vi "Practica_3.vi"() -> ()   [LabVIEW 2016]
uses:
  Control_1Enum.ctl
panel:
  out "String":string
  out "unsigned 8bit integer":u8
  out "Tab Control":T1(tab)
  out "Anuncios":u8(ring)
  in  "Boton_Aceptar_Contrasena":bool
  in  "Contrasena":string
  in  "Salir":bool
  out "Adeudo_Tarjeta":dbl
  out "Credito_Disponible":dbl
  in  "Estado_de_cuenta":bool
  in  "Depositos_otras_cuentas":bool
  in  "Donativos":bool
  in  "Compra_Tiempo_Aire":bool
  in  "Pago_Tarjeta_Credito":bool
  in  "Retirar Efectivo":bool
  in  "Regresar_1":bool
  in  "Retirar Efectivo 2":bool
  in  "Cantidad_a_Retirar":dbl min=0.0 max=10000.0
  out "Adeudo_Tarjeta 2":dbl
  out "Credito_Disponible 2":dbl
  in  "Regresar_2":bool
  in  "Monto_a_Pagar":dbl min=0.0 max=10000.0
  in  "Pago_Tarjeta_Credito 2":bool
  out "Adeudo_Tarjeta 3":dbl
  out "Credito_Disponible 3":dbl
  in  "Regresar_3":bool
  out "Adeudo_Tarjeta 4":dbl
  out "Credito_Disponible 4":dbl
  in  "Recargar_100":bool
  in  "Recargar_200":bool
  in  "Recargar_300":bool
  in  "Recargar_500":bool
  in  "Regresar_4":bool
  out "Adeudo_Tarjeta 5":dbl
  out "Credito_Disponible 5":dbl
  in  "Donar_100":bool
  in  "Donar_200":bool
  in  "Donar_300":bool
  in  "Donar_500":bool
  in  "Combo Box":string(combo)="World Vision Mexico"
  in  "Regresar_5":bool
  in  "Boton_Punto":bool
  out "String 2":string
  in  "Combo Box 2":string(combo)="Adrian Barba"
  out "Adeudo_Tarjeta 6":dbl
  out "Credito_Disponible 6":dbl
  in  "Boton_Aceptar":bool
  in  "Boton_Borrar":bool
  in  "Boton_9":bool
  in  "Boton_Limpiar":bool
  in  "Boton_6":bool
  in  "Boton_0":bool
  in  "Boton_3":bool
  in  "Boton_8":bool
  in  "Boton_7":bool
  in  "Boton_5":bool
  in  "Boton_4":bool
  in  "Boton_2":bool
  in  "Boton_1":bool
  in  "Regresar_6":bool
  out "Transacciones":string
  in  "Tarjeta":bool
  out "Led_Parpadeante":bool
  # "INGRESE SU CLAVE"
  # "Contraseña"
  # "Operaciones a Realizar"
  # "Retirar Credito"
  # "Pagar la Tarjeta"
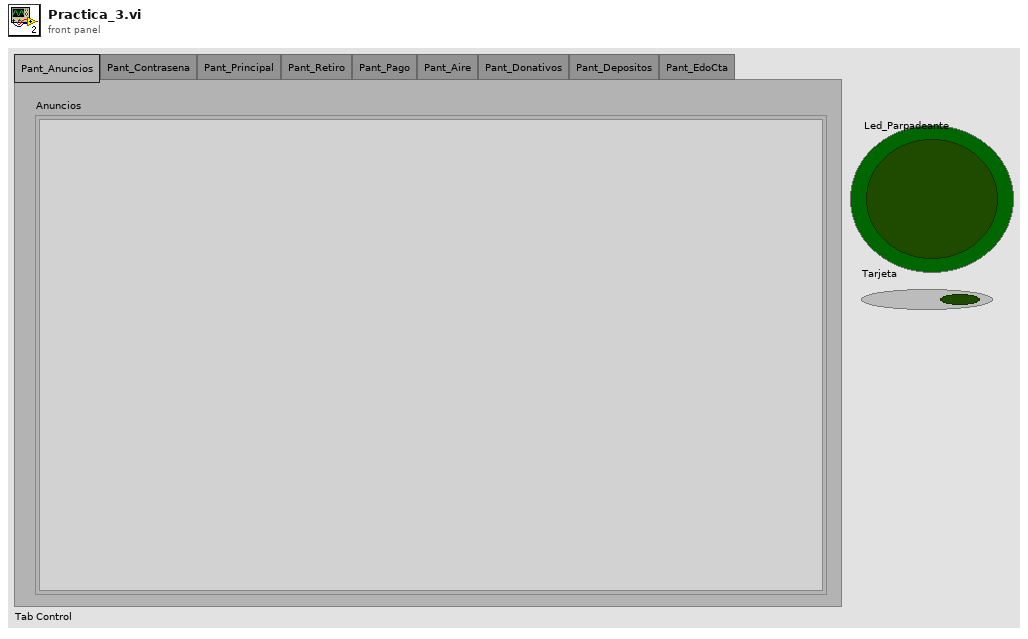
[diagram p1: front panel]
types:
  T1 = enum32{"Pant_Anuncios", "Pant_Contrasena", "Pant_Principal", "Pant_Retiro", "Pant_Pago", "Pant_Aire", "Pant_Donativos", "Pant_Depositos", "Pant_EdoCta"}
  T2 = typedef "Control_1Enum.ctl" = enum16{"Inicio", "Preguntar_Usuario", "Contrasena_valida", "Menu_Principal", "Menu_Retiro", "Menu_Pago", "Compra_TAire", "Donativos", "Depositos", "Estado_Cuenta"}
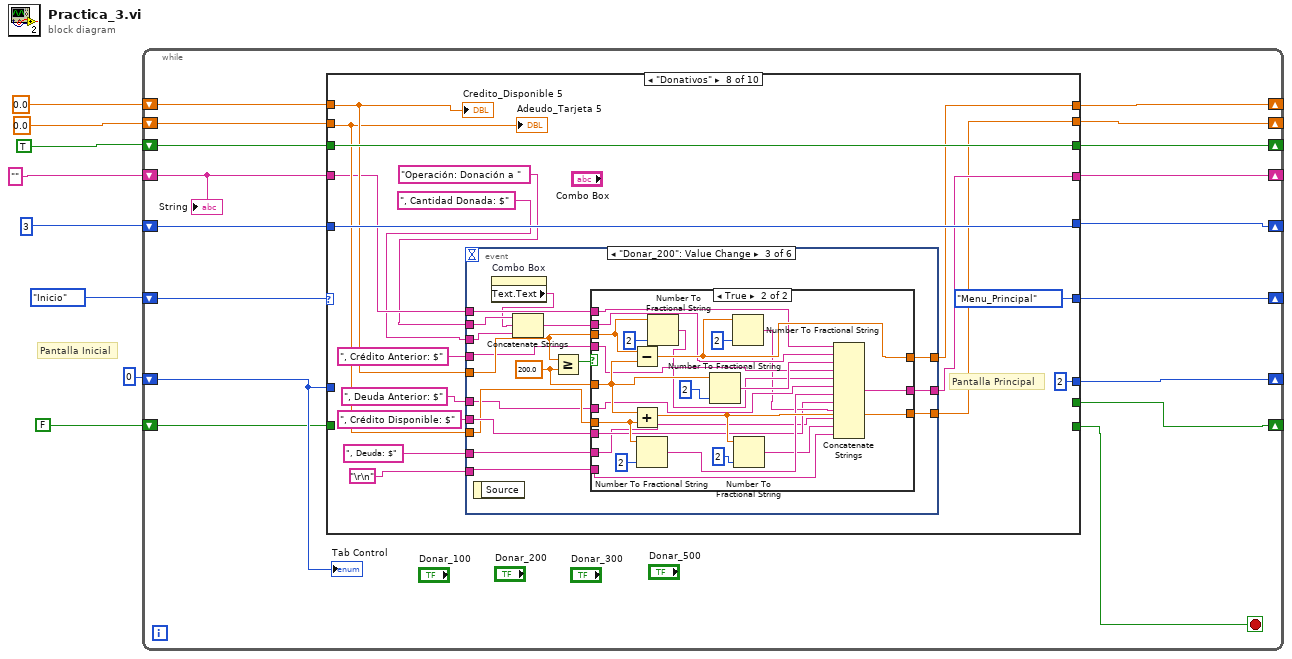
[diagram p0: block diagram]
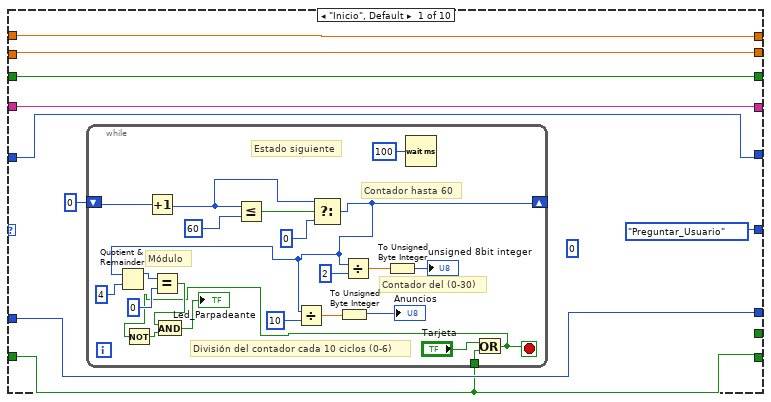
[diagram p2: hidden frame]
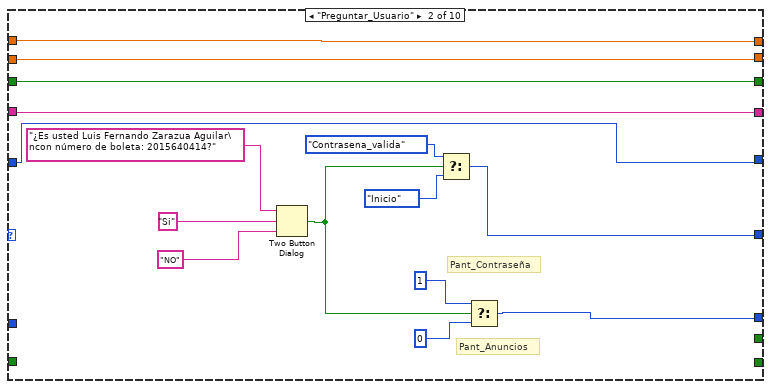
[diagram p3: hidden frame]
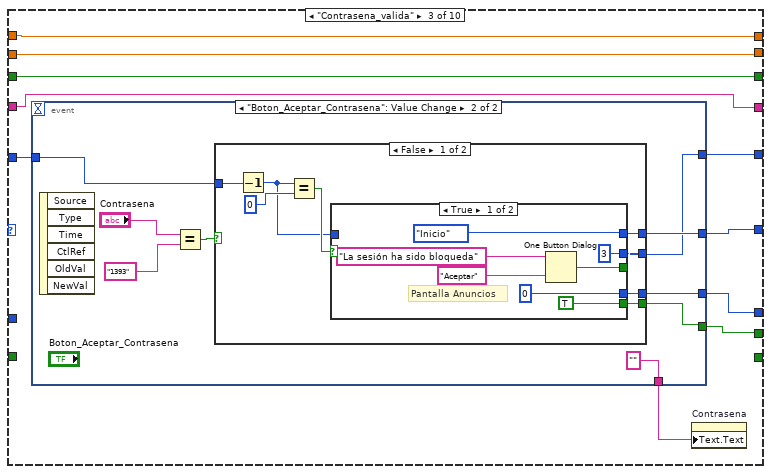
[diagram p4: hidden frame]
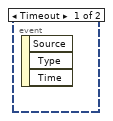
[diagram p5: hidden frame]
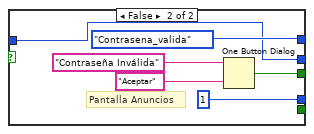
[diagram p6: hidden frame]
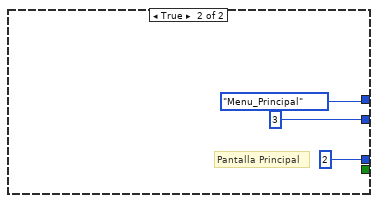
[diagram p7: hidden frame]
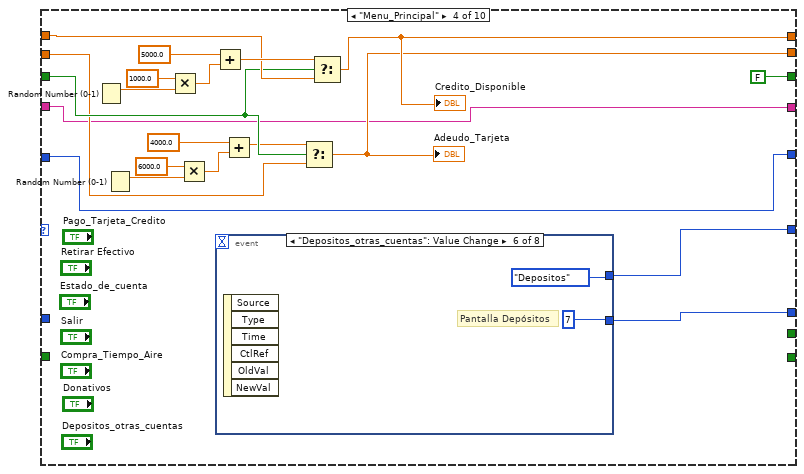
[diagram p8: hidden frame]
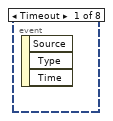
[diagram p9: hidden frame]
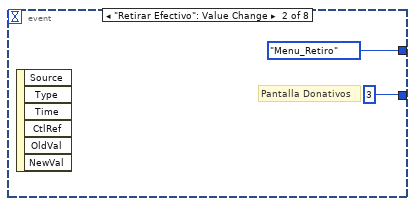
[diagram p10: hidden frame]
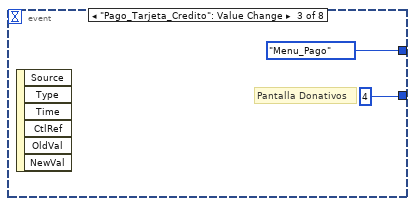
[diagram p11: hidden frame]
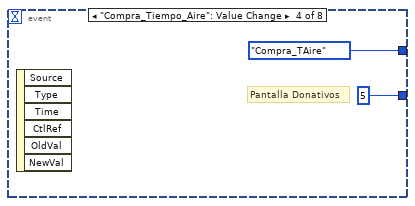
[diagram p12: hidden frame]
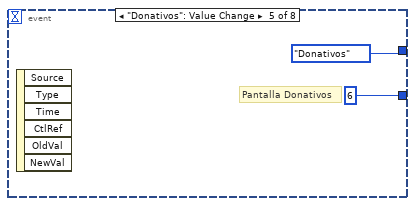
[diagram p13: hidden frame]
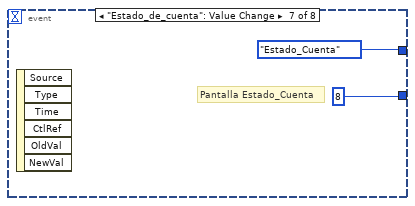
[diagram p14: hidden frame]
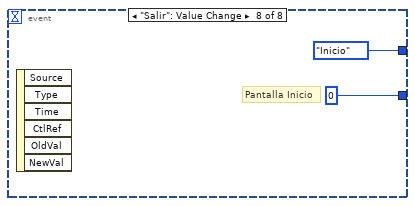
[diagram p15: hidden frame]
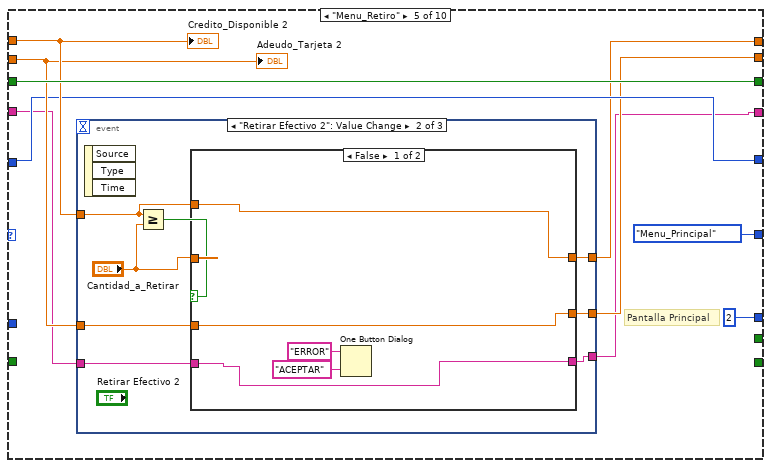
[diagram p16: hidden frame]
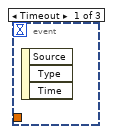
[diagram p17: hidden frame]
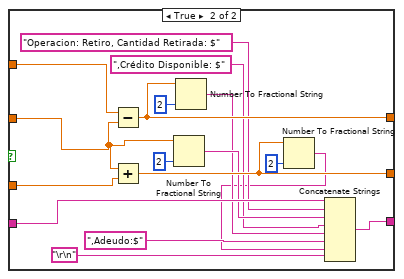
[diagram p18: hidden frame]
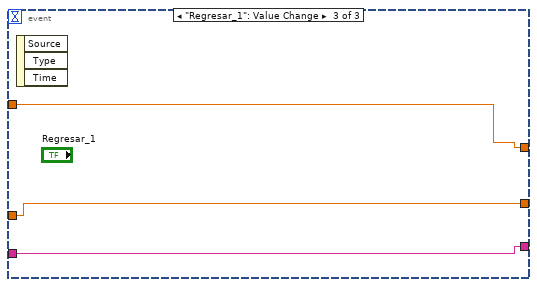
[diagram p19: hidden frame]
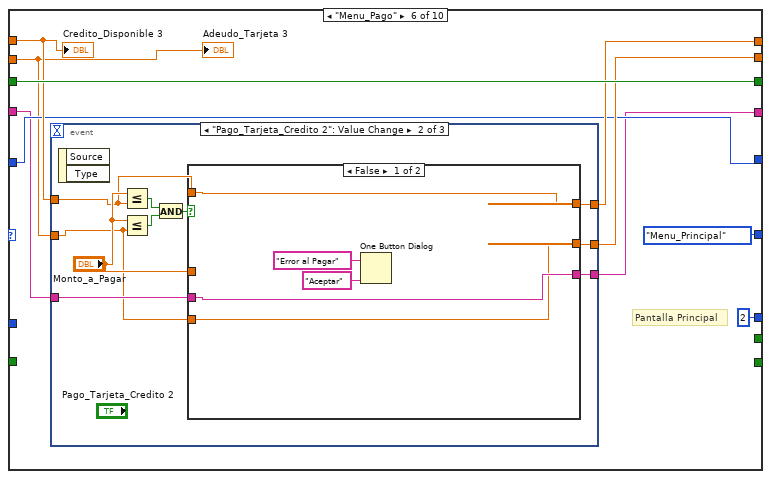
[diagram p20: hidden frame]
diagram:
  # "Pantalla Inicial"
  n1 = while {
    shift-right: [w22] -> _
    shift-left: Control_1Enum."Inicio" -> [w25]
    shift-right: [w23] -> _
    shift-left: u8 0 -> [w24]
    shift-right: [w20] -> _
    shift-left: TRUE -> [w21]
    shift-right: [w16] -> _
    shift-left: 0.0 -> [w19]
    shift-right: [w17] -> _
    shift-left: 0.0 -> [w18]
    shift-right: [w14] -> _
    shift-left: i8 3 -> [w15]
    shift-right: [w13] -> _
    shift-left: "" -> [w12]
    shift-right: [w9] -> _
    shift-left: FALSE -> [w11]
    stop <- w10 stop-if-true
    n2 = case shown="\"Donativos\"" w25 {
      tunnel: [w33 w66 w76 w117 u8 2 u8 2 u8 2 u8 2 w630 w798] -> w23
      tunnel: w24 -> [w33 _ _ _ _ _ _ _ _ _]
      tunnel: [Control_1Enum."Preguntar_Usuario" w64 w77 w118 Control_1Enum."Menu_Principal" Control_1Enum."Menu_Principal" Control_1Enum."Menu_Principal" Control_1Enum."Menu_Principal" w631 w799] -> w22
      tunnel: w21 -> [w31 w61 w79 w123 w158 w201 w252 w432 w629 w801]
      tunnel: [w31 w61 w79 FALSE w158 w201 w252 w432 w629 w801] -> w20
      tunnel: w19 -> [w29 w59 w81 w124 w156 w198 w248 w428 w621 w802]
      tunnel: w18 -> [w30 w60 w80 w121 w155 w192 w247 w427 w619 w803]
      tunnel: [w30 w60 w80 w119 w151 w196 w245 w418 w608 w803] -> w17
      tunnel: [w29 w59 w81 w120 w152 w197 w246 w420 w609 w802] -> w16
      tunnel: w15 -> [w28 w58 w78 w116 w153 w195 w249 w429 w628 w800]
      tunnel: [w28 w58 w75 w116 w153 w195 w249 w429 w628 w800] -> w14
      tunnel: w12 -> [w27 w57 w73 w115 w150 w194 w240 w421 w624 w797]
      tunnel: [w27 w57 w73 w115 w149 w193 w237 w419 w610 w796] -> w13
      tunnel: w11 -> [w26 _ _ _ _ _ _ _ _ _]
      tunnel: [w26 _ _ _ _ _ _ _ _ _] -> w10
      tunnel: [_ _ w72 _ _ _ _ _ _ _] -> w9
      frame "Inicio", Default {
        (unwired) u8 0
        n3 = while {
          shift-right: [w44] -> _
          shift-left: i8 0 -> [w55]
          tunnel: w26 -> [w35]
          stop <- w37 stop-if-true
          # "Contador del (0-30)"
          # "Módulo"
          # "División del contador cada 10 ciclos (0-6)"
          # "Contador hasta 60"
          # "Estado siguiente"
          n4 = Increment(x=w55) -> (x+1=w52:i8)
          n5 = Less Or Equal?(x=w52, y=i8 60) -> (x <= y?=w53:bool)
          n6 = Select(t=w52, s=w53, f=i8 0) -> (s? t:f=w44:i8)
          n7 = Quotient & Remainder(x=w44, y=i8 4) -> (x-y*floor(x/y)=w42:i8)  [unwired: 1 out]
          n8 = Equal?(x=w42, y=i8 0) -> (x = y?=w39:bool)
          n9 = Divide(x=w44, y=i8 10) -> (x/y=w48:dbl)
          n10 = To Unsigned Byte Integer(number=w48) -> (unsigned 8bit integer=→"Anuncios":u8)
          n11 = Divide(x=w44, y=i8 2) -> (x/y=w46:dbl)
          n12 = To Unsigned Byte Integer(number=w46) -> (unsigned 8bit integer=→"unsigned 8bit integer":u8)
          n13 = Wait (ms)(milliseconds to wait=u32 100) -> ()  [unwired: 1 out]
          n14 = Or(x="Tarjeta", y=w35) -> (x .or. y?=w37:bool)
          n15 = Not(x=w37) -> (.not. x?=w38:bool)
          n16 = And(x=w39, y=w38) -> (x .and. y?=→"Led_Parpadeante":bool)
        }
      }
      frame "Preguntar_Usuario" {
        # "Pant_Anuncios"
        # "Pant_Contraseña"
        n17 = Two Button Dialog(message="¿Es usted Luis Fernando Zarazua Aguilar\ncon número de boleta: 2015640414?", 1:"NO" ("F button name (\"Cancel\")"), 2:"Si" ("T button name (\"OK\")")) -> (T button?=w65:bool)
        n18 = Select(t=Control_1Enum."Contrasena_valida", s=w65, f=Control_1Enum."Inicio") -> (s? t:f=w64:T2)
        n19 = Select(t=u8 1, s=w65, f=0) -> (s? t:f=w66:i32)
      }
      frame "Contrasena_valida" {
        n20 = event shown="[1] \"Boton_Aceptar_Contrasena\": Value Change" {
          selector: _ -> [_ _]
          dyn-events: _ -> [_ _]
          timeout: _ -> [_ _]
          tunnel: w78 -> [_ w87]
          tunnel: [_ w86] -> w77
          tunnel: [_ w85] -> w76
          tunnel: [_ w84] -> w75
          tunnel: [_ "" ("Label.Text")] -> w74
          tunnel: [_ w82] -> w72
          event Timeout {
            n21 = event-data() -> ()  [unwired: 1 in, 3 out]
          }
          event "Boton_Aceptar_Contrasena": Value Change {
            n22 = event-data() -> ()  [unwired: 1 in, 6 out]
            n23 = Equal?(x="Contrasena", y="1393") -> (x = y?=w88:bool)
            n24 = case shown="False" w88 {
              tunnel: w87 -> [w93 _]
              tunnel: [w96 Control_1Enum."Menu_Principal"] -> w86
              tunnel: [w95 u8 2] -> w85
              tunnel: [w94 i8 3] -> w84
              tunnel: [w91 _] -> w82
              frame False {
                n25 = Decrement(x=w93) -> (x-1=w92:i8)
                n26 = Equal?(x=w92, y=i8 0) -> (x = y?=w97:bool)
                n27 = case shown="True" w97 {
                  tunnel: [Control_1Enum."Inicio" Control_1Enum."Contrasena_valida"] -> w96
                  tunnel: [u8 0 u8 1] -> w95
                  tunnel: [w101 w107] -> _
                  tunnel: [i8 3 w106] -> w94
                  tunnel: w92 -> [_ w106]
                  tunnel: [TRUE _] -> w91
                  frame True {
                    # "Pantalla Anuncios"
                    n28 = One Button Dialog(message="La sesión ha sido bloqueda", button name ("OK")="Aceptar") -> (true=w101:bool)
                  }
                  frame False {
                    # "Pantalla Anuncios"
                    n29 = One Button Dialog(message="Contraseña Inválida", button name ("OK")="Aceptar") -> (true=w107:bool)
                  }
                }
              }
              frame True {
                # "Pantalla Principal"
              }
            }
          }
        }
        n30 = property on="Contrasena" class="Str"("Text.Text"=w74) -> ()  [unwired: 2 in, 2 out]
      }
      frame "Menu_Principal" {
        n31 = Random Number (0-1)() -> (number: 0 to 1=w134:dbl)
        n32 = Random Number (0-1)() -> (number: 0 to 1=w130:dbl)
        n33 = Multiply(x=1000.0, y=w134) -> (x*y=w131:dbl)
        n34 = Multiply(x=6000.0, y=w130) -> (x*y=w127:dbl)
        n35 = Add(x=5000.0, y=w131) -> (x+y=w126:dbl)
        n36 = event shown="[5] \"Depositos_otras_cuentas\": Value Change" {
          selector: _ -> [_ _ _ _ _ _ _ _]
          dyn-events: _ -> [_ _ _ _ _ _ _ _]
          timeout: _ -> [_ _ _ _ _ _ _ _]
          tunnel: [_ Control_1Enum."Menu_Retiro" Control_1Enum."Menu_Pago" Control_1Enum."Compra_TAire" Control_1Enum."Donativos" Control_1Enum."Depositos" Control_1Enum."Estado_Cuenta" Control_1Enum."Inicio"] -> w118
          tunnel: [_ u8 3 u8 4 u8 5 u8 6 u8 7 u8 8 u8 0] -> w117
          event Timeout {
            n37 = event-data() -> ()  [unwired: 1 in, 3 out]
          }
          event "Retirar Efectivo": Value Change {
            # "Pantalla Donativos"
            n38 = event-data() -> ()  [unwired: 1 in, 6 out]
          }
          event "Pago_Tarjeta_Credito": Value Change {
            # "Pantalla Donativos"
            n39 = event-data() -> ()  [unwired: 1 in, 6 out]
          }
          event "Compra_Tiempo_Aire": Value Change {
            # "Pantalla Donativos"
            n40 = event-data() -> ()  [unwired: 1 in, 6 out]
          }
          event "Donativos": Value Change {
            # "Pantalla Donativos"
            n41 = event-data() -> ()  [unwired: 1 in, 6 out]
          }
          event "Depositos_otras_cuentas": Value Change {
            # "Pantalla Depósitos"
            n42 = event-data() -> ()  [unwired: 1 in, 6 out]
          }
          event "Estado_de_cuenta": Value Change {
            # "Pantalla Estado_Cuenta"
            n43 = event-data() -> ()  [unwired: 1 in, 6 out]
          }
          event "Salir": Value Change {
            # "Pantalla Inicio"
            n44 = event-data() -> ()  [unwired: 1 in, 6 out]
          }
        }
        n45 = Add(x=4000.0, y=w127) -> (x+y=w122:dbl)
        n46 = Select(t=w122, s=w123, f=w121) -> (s? t:f=w119:dbl)
        "Adeudo_Tarjeta" <- w119
        n47 = Select(t=w126, s=w123, f=w124) -> (s? t:f=w120:dbl)
        "Credito_Disponible" <- w120
      }
      frame "Menu_Retiro" {
        # "Pantalla Principal"
        n48 = event shown="[1] \"Retirar Efectivo 2\": Value Change" {
          selector: _ -> [_ _ _]
          dyn-events: _ -> [_ _ _]
          timeout: _ -> [_ _ _]
          tunnel: w156 -> [_ w159 w191]
          tunnel: w155 -> [_ w165 w189]
          tunnel: [_ w163 w191] -> w152
          tunnel: [_ w162 w189] -> w151
          tunnel: w150 -> [_ w161 w190]
          tunnel: [_ w160 w190] -> w149
          event Timeout {
            n49 = event-data() -> ()  [unwired: 1 in, 3 out]
          }
          event "Retirar Efectivo 2": Value Change {
            n50 = event-data() -> ()  [unwired: 1 in, 3 out]
            n51 = Greater Or Equal?(x=w159, y="Cantidad_a_Retirar") -> (x >= y?=w164:bool)
            n52 = case shown="False" w164 {
              tunnel: "Cantidad_a_Retirar" -> [_ w179]
              tunnel: w165 -> [w169 w188]
              tunnel: w159 -> [w168 w187]
              tunnel: [w169 w183] -> w162
              tunnel: [w168 w182] -> w163
              tunnel: w161 -> [w167 w185]
              tunnel: [w167 w186] -> w160
              frame False {
                n53 = One Button Dialog(message="ERROR", button name ("OK")="ACEPTAR") -> ()  [unwired: 1 out]
              }
              frame True {
                n54 = Subtract(x=w187, y=w179) -> (x-y=w182:dbl)
                n55 = Add(x=w179, y=w188) -> (x+y=w183:dbl)
                n56 = Number To Fractional String(number=w179, precision (6)=i16 2 ("width (-)")) -> (F-format string=w177:string)  [unwired: 2 in]
                n57 = Number To Fractional String(number=w182, precision (6)=i16 2 ("width (-)")) -> (F-format string=w175:string)  [unwired: 2 in]
                n58 = Number To Fractional String(number=w183, precision (6)=i16 2 ("width (-)")) -> (F-format string=w173:string)  [unwired: 2 in]
                n59 = Concatenate Strings(w185, "Operacion: Retiro, Cantidad Retirada: $" ("string"), w177, ",Crédito Disponible: $" ("string"), w175, ",Adeudo:$" ("string"), w173, "\r\n") -> (w186:string)
              }
            }
          }
          event "Regresar_1": Value Change {
            n60 = event-data() -> ()  [unwired: 1 in, 3 out]
          }
        }
        "Credito_Disponible 2" <- w156
        "Adeudo_Tarjeta 2" <- w155
      }
      frame "Menu_Pago" {
        # "Pantalla Principal"
        n61 = event shown="[1] \"Pago_Tarjeta_Credito 2\": Value Change" {
          selector: _ -> [_ _ _]
          dyn-events: _ -> [_ _ _]
          timeout: _ -> [_ _ _]
          tunnel: w198 -> [_ w207 w236]
          tunnel: [_ w206 w236] -> w197
          tunnel: [_ w205 w235] -> w196
          tunnel: [_ w204 w234] -> w193
          tunnel: w194 -> [_ w203 w234]
          tunnel: w192 -> [_ w202 w235]
          event Timeout {
            n62 = event-data() -> ()  [unwired: 1 in, 3 out]
          }
          event "Pago_Tarjeta_Credito 2": Value Change {
            n63 = event-data() -> ()  [unwired: 1 in, 2 out]
            n64 = Less Or Equal?(x="Monto_a_Pagar", y=w207) -> (x <= y?=w211:bool)
            n65 = Less Or Equal?(x="Monto_a_Pagar", y=w202) -> (x <= y?=w210:bool)
            n66 = And(x=w211, y=w210) -> (x .and. y?=w209:bool)
            n67 = case shown="False" w209 {
              tunnel: "Monto_a_Pagar" -> [_ w223]
              tunnel: [w212 w221] -> w205
              tunnel: [w213 w222] -> w206
              tunnel: w207 -> [w213 w224]
              tunnel: [w214 w220] -> w204
              tunnel: w203 -> [w214 w219]
              tunnel: w202 -> [w212 w217]
              frame False {
                n68 = One Button Dialog(message="Error al Pagar", button name ("OK")="Aceptar") -> ()  [unwired: 1 out]
              }
              frame True {
                n69 = Add(x=w224, y=w223) -> (x+y=w222:dbl)
                n70 = Subtract(x=w217, y=w223) -> (x-y=w221:dbl)
                n71 = Number To Fractional String(number=w223, precision (6)=i16 2 ("width (-)")) -> (F-format string=w230:string)  [unwired: 2 in]
                n72 = Number To Fractional String(number=w222, precision (6)=i16 2 ("width (-)")) -> (F-format string=w228:string)  [unwired: 2 in]
                n73 = Number To Fractional String(number=w221, precision (6)=i16 2 ("width (-)")) -> (F-format string=w226:string)  [unwired: 2 in]
                n74 = Concatenate Strings(w219, "Operacion: Pago de Tarjeta, Cantidad Ingresada: $" ("string"), w230, ",Crédito Disponible: $" ("string"), w228, ",Adeudo:$" ("string"), w226, "\r\n") -> (w220:string)
              }
            }
          }
          event "Regresar_2": Value Change {
            n75 = event-data() -> ()  [unwired: 1 in, 2 out]
          }
        }
        "Adeudo_Tarjeta 3" <- w192
        "Credito_Disponible 3" <- w198
      }
      frame "Compra_TAire" {
        # "Pantalla Principal"
        n76 = event shown="[1] \"Recargar_100\": Value Change" {
          selector: _ -> [_ _ _ _ _ _]
          dyn-events: _ -> [_ _ _ _ _ _]
          timeout: _ -> [_ _ _ _ _ _]
          tunnel: w248 -> [_ w265 w305 w345 w385 w414]
          tunnel: w247 -> [_ w264 w304 w344 w384 w413]
          tunnel: [_ w262 w302 w342 w382 w414] -> w246
          tunnel: [_ w261 w301 w341 w381 w413] -> w245
          tunnel: "\r\n" -> [_ w254 w294 w334 w374 _]
          tunnel: ", Deuda: $" -> [_ w255 w295 w335 w375 _]
          tunnel: ", Crédito Disponible: $" -> [_ w256 w296 w336 w376 _]
          tunnel: ", Deuda Anterior: $" -> [_ w257 w297 w337 w377 _]
          tunnel: ", Crédito Anterior: $" -> [_ w258 w298 w338 w378 _]
          tunnel: "Operación: Recarga de Tiempo Aire, Cantidad Recargada: $" -> [_ w259 w299 w339 w379 _]
          tunnel: w240 -> [_ w260 w300 w340 w380 w415]
          tunnel: [_ w253 w293 w333 w373 w415] -> w237
          event Timeout {
            n77 = event-data() -> ()  [unwired: 1 in, 3 out]
          }
          event "Recargar_100": Value Change {
            w263 = 100.0 ("y")
            n78 = event-data() -> ()  [unwired: 1 in, 1 out]
            n79 = Greater Or Equal?(x=w265, y=w263) -> (x >= y?=w266:bool)
            n80 = case shown="True" w266 {
              tunnel: [w267 w290] -> w261
              tunnel: [w268 w287] -> w262
              tunnel: w265 -> [w268 w285]
              tunnel: w264 -> [w267 w283]
              tunnel: w263 -> [_ w291]
              tunnel: w260 -> [w269 w286]
              tunnel: w259 -> [_ w281]
              tunnel: w258 -> [_ w279]
              tunnel: w257 -> [_ w277]
              tunnel: w256 -> [_ w274]
              tunnel: w255 -> [_ w273]
              tunnel: w254 -> [_ w271]
              tunnel: [w269 w270] -> w253
              frame False {
              }
              frame True {
                n81 = Subtract(x=w285, y=w291) -> (x-y=w287:dbl)
                n82 = Add(x=w291, y=w283) -> (x+y=w290:dbl)
                n83 = Number To Fractional String(number=w283, precision (6)=i16 2) -> (F-format string=w276:string)  [unwired: 2 in]
                n84 = Number To Fractional String(number=w285, precision (6)=i16 2) -> (F-format string=w278:string)  [unwired: 2 in]
                n85 = Number To Fractional String(number=w291, precision (6)=i16 2) -> (F-format string=w280:string)  [unwired: 2 in]
                n86 = Number To Fractional String(number=w287, precision (6)=i16 2) -> (F-format string=w275:string)  [unwired: 2 in]
                n87 = Number To Fractional String(number=w290, precision (6)=i16 2) -> (F-format string=w272:string)  [unwired: 2 in]
                n88 = Concatenate Strings(w286, w281, w280, w279, w278, w277, w276, w274, w275, w273, w272, w271) -> (w270:string)
              }
            }
          }
          event "Recargar_200": Value Change {
            w303 = 200.0 ("y")
            n89 = event-data() -> ()  [unwired: 1 in, 1 out]
            n90 = Greater Or Equal?(x=w305, y=w303) -> (x >= y?=w306:bool)
            n91 = case shown="True" w306 {
              tunnel: [w307 w330] -> w301
              tunnel: [w308 w327] -> w302
              tunnel: w305 -> [w308 w325]
              tunnel: w304 -> [w307 w323]
              tunnel: w303 -> [_ w331]
              tunnel: w300 -> [w309 w326]
              tunnel: w299 -> [_ w321]
              tunnel: w298 -> [_ w319]
              tunnel: w297 -> [_ w317]
              tunnel: w296 -> [_ w314]
              tunnel: w295 -> [_ w313]
              tunnel: w294 -> [_ w311]
              tunnel: [w309 w310] -> w293
              frame False {
              }
              frame True {
                n92 = Subtract(x=w325, y=w331) -> (x-y=w327:dbl)
                n93 = Add(x=w331, y=w323) -> (x+y=w330:dbl)
                n94 = Number To Fractional String(number=w323, precision (6)=i16 2) -> (F-format string=w316:string)  [unwired: 2 in]
                n95 = Number To Fractional String(number=w325, precision (6)=i16 2) -> (F-format string=w318:string)  [unwired: 2 in]
                n96 = Number To Fractional String(number=w331, precision (6)=i16 2) -> (F-format string=w320:string)  [unwired: 2 in]
                n97 = Number To Fractional String(number=w327, precision (6)=i16 2) -> (F-format string=w315:string)  [unwired: 2 in]
                n98 = Number To Fractional String(number=w330, precision (6)=i16 2) -> (F-format string=w312:string)  [unwired: 2 in]
                n99 = Concatenate Strings(w326, w321, w320, w319, w318, w317, w316, w314, w315, w313, w312, w311) -> (w310:string)
              }
            }
          }
          event "Recargar_300": Value Change {
            w343 = 300.0 ("y")
            n100 = event-data() -> ()  [unwired: 1 in, 1 out]
            n101 = Greater Or Equal?(x=w345, y=w343) -> (x >= y?=w346:bool)
            n102 = case shown="True" w346 {
              tunnel: [w347 w370] -> w341
              tunnel: [w348 w367] -> w342
              tunnel: w345 -> [w348 w365]
              tunnel: w344 -> [w347 w363]
              tunnel: w343 -> [_ w371]
              tunnel: w340 -> [w349 w366]
              tunnel: w339 -> [_ w361]
              tunnel: w338 -> [_ w359]
              tunnel: w337 -> [_ w357]
              tunnel: w336 -> [_ w354]
              tunnel: w335 -> [_ w353]
              tunnel: w334 -> [_ w351]
              tunnel: [w349 w350] -> w333
              frame False {
              }
              frame True {
                n103 = Subtract(x=w365, y=w371) -> (x-y=w367:dbl)
                n104 = Add(x=w371, y=w363) -> (x+y=w370:dbl)
                n105 = Number To Fractional String(number=w363, precision (6)=i16 2) -> (F-format string=w356:string)  [unwired: 2 in]
                n106 = Number To Fractional String(number=w365, precision (6)=i16 2) -> (F-format string=w358:string)  [unwired: 2 in]
                n107 = Number To Fractional String(number=w371, precision (6)=i16 2) -> (F-format string=w360:string)  [unwired: 2 in]
                n108 = Number To Fractional String(number=w367, precision (6)=i16 2) -> (F-format string=w355:string)  [unwired: 2 in]
                n109 = Number To Fractional String(number=w370, precision (6)=i16 2) -> (F-format string=w352:string)  [unwired: 2 in]
                n110 = Concatenate Strings(w366, w361, w360, w359, w358, w357, w356, w354, w355, w353, w352, w351) -> (w350:string)
              }
            }
          }
          event "Recargar_500": Value Change {
            w383 = 500.0 ("y")
            n111 = event-data() -> ()  [unwired: 1 in, 1 out]
            n112 = Greater Or Equal?(x=w385, y=w383) -> (x >= y?=w386:bool)
            n113 = case shown="True" w386 {
              tunnel: [w387 w410] -> w381
              tunnel: [w388 w407] -> w382
              tunnel: w385 -> [w388 w405]
              tunnel: w384 -> [w387 w403]
              tunnel: w383 -> [_ w411]
              tunnel: w380 -> [w389 w406]
              tunnel: w379 -> [_ w401]
              tunnel: w378 -> [_ w399]
              tunnel: w377 -> [_ w397]
              tunnel: w376 -> [_ w394]
              tunnel: w375 -> [_ w393]
              tunnel: w374 -> [_ w391]
              tunnel: [w389 w390] -> w373
              frame False {
              }
              frame True {
                n114 = Subtract(x=w405, y=w411) -> (x-y=w407:dbl)
                n115 = Add(x=w411, y=w403) -> (x+y=w410:dbl)
                n116 = Number To Fractional String(number=w403, precision (6)=i16 2) -> (F-format string=w396:string)  [unwired: 2 in]
                n117 = Number To Fractional String(number=w405, precision (6)=i16 2) -> (F-format string=w398:string)  [unwired: 2 in]
                n118 = Number To Fractional String(number=w411, precision (6)=i16 2) -> (F-format string=w400:string)  [unwired: 2 in]
                n119 = Number To Fractional String(number=w407, precision (6)=i16 2) -> (F-format string=w395:string)  [unwired: 2 in]
                n120 = Number To Fractional String(number=w410, precision (6)=i16 2) -> (F-format string=w392:string)  [unwired: 2 in]
                n121 = Concatenate Strings(w406, w401, w400, w399, w398, w397, w396, w394, w395, w393, w392, w391) -> (w390:string)
              }
            }
          }
          event "Regresar_3": Value Change {
            n122 = event-data() -> ()  [unwired: 1 in, 1 out]
          }
        }
        "Credito_Disponible 4" <- w248
        "Adeudo_Tarjeta 4" <- w247
      }
      frame "Donativos" {
        # "Pantalla Principal"
        n123 = event shown="[2] \"Donar_200\": Value Change" {
          selector: _ -> [_ _ _ _ _ _]
          dyn-events: _ -> [_ _ _ _ _ _]
          timeout: _ -> [_ _ _ _ _ _]
          tunnel: w428 -> [_ w442 w485 w528 w571 w606]
          tunnel: w427 -> [_ w444 w487 w530 w573 w605]
          tunnel: "\r\n" -> [_ w447 w490 w533 w576 _]
          tunnel: ", Deuda: $" -> [_ w446 w489 w532 w575 _]
          tunnel: ", Crédito Disponible: $" -> [_ w445 w488 w531 w574 _]
          tunnel: ", Deuda Anterior: $" -> [_ w443 w486 w529 w572 _]
          tunnel: ", Crédito Anterior: $" -> [_ w441 w484 w527 w570 _]
          tunnel: w421 -> [_ w440 w483 w526 w569 w607]
          tunnel: [_ w439 w482 w525 w568 w606] -> w420
          tunnel: [_ w438 w481 w524 w567 w607] -> w419
          tunnel: [_ w437 w480 w523 w566 w605] -> w418
          tunnel: "Operación: Donación a " -> [_ w435 w478 w521 w564 _]
          tunnel: ", Cantidad Donada: $" -> [_ w434 w477 w520 w563 _]
          event Timeout {
            n124 = event-data() -> ()  [unwired: 1 in, 3 out]
          }
          event "Donar_100": Value Change {
            w448 = 100.0 ("y")
            n125 = event-data() -> ()  [unwired: 1 in, 1 out]
            n126 = property on="Combo Box" class="CmbBox"() -> ("Text.Text"=w433:string)  [unwired: 2 in, 2 out]
            n127 = Concatenate Strings(w435, w433, w434) -> (w436:string)
            n128 = Greater Or Equal?(x=w442, y=w448) -> (x >= y?=w449:bool)
            n129 = case shown="True" w449 {
              tunnel: [w450 w473] -> w437
              tunnel: [w451 w470] -> w439
              tunnel: w442 -> [w451 w468]
              tunnel: w444 -> [w450 w466]
              tunnel: w448 -> [_ w474]
              tunnel: w440 -> [w452 w469]
              tunnel: w436 -> [_ w464]
              tunnel: w441 -> [_ w462]
              tunnel: w443 -> [_ w460]
              tunnel: w445 -> [_ w457]
              tunnel: w446 -> [_ w456]
              tunnel: w447 -> [_ w454]
              tunnel: [w452 w453] -> w438
              frame False {
              }
              frame True {
                n130 = Subtract(x=w468, y=w474) -> (x-y=w470:dbl)
                n131 = Add(x=w474, y=w466) -> (x+y=w473:dbl)
                n132 = Number To Fractional String(number=w466, precision (6)=i16 2) -> (F-format string=w459:string)  [unwired: 2 in]
                n133 = Number To Fractional String(number=w468, precision (6)=i16 2) -> (F-format string=w461:string)  [unwired: 2 in]
                n134 = Number To Fractional String(number=w474, precision (6)=i16 2) -> (F-format string=w463:string)  [unwired: 2 in]
                n135 = Number To Fractional String(number=w470, precision (6)=i16 2) -> (F-format string=w458:string)  [unwired: 2 in]
                n136 = Number To Fractional String(number=w473, precision (6)=i16 2) -> (F-format string=w455:string)  [unwired: 2 in]
                n137 = Concatenate Strings(w469, w464, w463, w462, w461, w460, w459, w457, w458, w456, w455, w454) -> (w453:string)
              }
            }
          }
          event "Donar_200": Value Change {
            w491 = 200.0 ("y")
            n138 = event-data() -> ()  [unwired: 1 in, 1 out]
            n139 = property on="Combo Box" class="CmbBox"() -> ("Text.Text"=w476:string)  [unwired: 2 in, 2 out]
            n140 = Concatenate Strings(w478, w476, w477) -> (w479:string)
            n141 = Greater Or Equal?(x=w485, y=w491) -> (x >= y?=w492:bool)
            n142 = case shown="True" w492 {
              tunnel: [w493 w516] -> w480
              tunnel: [w494 w513] -> w482
              tunnel: w485 -> [w494 w511]
              tunnel: w487 -> [w493 w509]
              tunnel: w491 -> [_ w517]
              tunnel: w483 -> [w495 w512]
              tunnel: w479 -> [_ w507]
              tunnel: w484 -> [_ w505]
              tunnel: w486 -> [_ w503]
              tunnel: w488 -> [_ w500]
              tunnel: w489 -> [_ w499]
              tunnel: w490 -> [_ w497]
              tunnel: [w495 w496] -> w481
              frame False {
              }
              frame True {
                n143 = Subtract(x=w511, y=w517) -> (x-y=w513:dbl)
                n144 = Add(x=w517, y=w509) -> (x+y=w516:dbl)
                n145 = Number To Fractional String(number=w509, precision (6)=i16 2) -> (F-format string=w502:string)  [unwired: 2 in]
                n146 = Number To Fractional String(number=w511, precision (6)=i16 2) -> (F-format string=w504:string)  [unwired: 2 in]
                n147 = Number To Fractional String(number=w517, precision (6)=i16 2) -> (F-format string=w506:string)  [unwired: 2 in]
                n148 = Number To Fractional String(number=w513, precision (6)=i16 2) -> (F-format string=w501:string)  [unwired: 2 in]
                n149 = Number To Fractional String(number=w516, precision (6)=i16 2) -> (F-format string=w498:string)  [unwired: 2 in]
                n150 = Concatenate Strings(w512, w507, w506, w505, w504, w503, w502, w500, w501, w499, w498, w497) -> (w496:string)
              }
            }
          }
          event "Donar_300": Value Change {
            w534 = 300.0 ("y")
            n151 = event-data() -> ()  [unwired: 1 in, 1 out]
            n152 = property on="Combo Box" class="CmbBox"() -> ("Text.Text"=w519:string)  [unwired: 2 in, 2 out]
            n153 = Concatenate Strings(w521, w519, w520) -> (w522:string)
            n154 = Greater Or Equal?(x=w528, y=w534) -> (x >= y?=w535:bool)
            n155 = case shown="True" w535 {
              tunnel: [w536 w559] -> w523
              tunnel: [w537 w556] -> w525
              tunnel: w528 -> [w537 w554]
              tunnel: w530 -> [w536 w552]
              tunnel: w534 -> [_ w560]
              tunnel: w526 -> [w538 w555]
              tunnel: w522 -> [_ w550]
              tunnel: w527 -> [_ w548]
              tunnel: w529 -> [_ w546]
              tunnel: w531 -> [_ w543]
              tunnel: w532 -> [_ w542]
              tunnel: w533 -> [_ w540]
              tunnel: [w538 w539] -> w524
              frame False {
              }
              frame True {
                n156 = Subtract(x=w554, y=w560) -> (x-y=w556:dbl)
                n157 = Add(x=w560, y=w552) -> (x+y=w559:dbl)
                n158 = Number To Fractional String(number=w552, precision (6)=i16 2) -> (F-format string=w545:string)  [unwired: 2 in]
                n159 = Number To Fractional String(number=w554, precision (6)=i16 2) -> (F-format string=w547:string)  [unwired: 2 in]
                n160 = Number To Fractional String(number=w560, precision (6)=i16 2) -> (F-format string=w549:string)  [unwired: 2 in]
                n161 = Number To Fractional String(number=w556, precision (6)=i16 2) -> (F-format string=w544:string)  [unwired: 2 in]
                n162 = Number To Fractional String(number=w559, precision (6)=i16 2) -> (F-format string=w541:string)  [unwired: 2 in]
                n163 = Concatenate Strings(w555, w550, w549, w548, w547, w546, w545, w543, w544, w542, w541, w540) -> (w539:string)
              }
            }
          }
          event "Donar_500": Value Change {
            w577 = 500.0 ("y")
            n164 = event-data() -> ()  [unwired: 1 in, 1 out]
            n165 = property on="Combo Box" class="CmbBox"() -> ("Text.Text"=w562:string)  [unwired: 2 in, 2 out]
            n166 = Concatenate Strings(w564, w562, w563) -> (w565:string)
            n167 = Greater Or Equal?(x=w571, y=w577) -> (x >= y?=w578:bool)
            n168 = case shown="True" w578 {
              tunnel: [w579 w602] -> w566
              tunnel: [w580 w599] -> w568
              tunnel: w571 -> [w580 w597]
              tunnel: w573 -> [w579 w595]
              tunnel: w577 -> [_ w603]
              tunnel: w569 -> [w581 w598]
              tunnel: w565 -> [_ w593]
              tunnel: w570 -> [_ w591]
              tunnel: w572 -> [_ w589]
              tunnel: w574 -> [_ w586]
              tunnel: w575 -> [_ w585]
              tunnel: w576 -> [_ w583]
              tunnel: [w581 w582] -> w567
              frame False {
              }
              frame True {
                n169 = Subtract(x=w597, y=w603) -> (x-y=w599:dbl)
                n170 = Add(x=w603, y=w595) -> (x+y=w602:dbl)
                n171 = Number To Fractional String(number=w595, precision (6)=i16 2) -> (F-format string=w588:string)  [unwired: 2 in]
                n172 = Number To Fractional String(number=w597, precision (6)=i16 2) -> (F-format string=w590:string)  [unwired: 2 in]
                n173 = Number To Fractional String(number=w603, precision (6)=i16 2) -> (F-format string=w592:string)  [unwired: 2 in]
                n174 = Number To Fractional String(number=w599, precision (6)=i16 2) -> (F-format string=w587:string)  [unwired: 2 in]
                n175 = Number To Fractional String(number=w602, precision (6)=i16 2) -> (F-format string=w584:string)  [unwired: 2 in]
                n176 = Concatenate Strings(w598, w593, w592, w591, w590, w589, w588, w586, w587, w585, w584, w583) -> (w582:string)
              }
            }
          }
          event "Regresar_4": Value Change {
            n177 = event-data() -> ()  [unwired: 1 in, 2 out]
          }
        }
        "Credito_Disponible 5" <- w428
        "Adeudo_Tarjeta 5" <- w427
      }
      frame "Depositos" {
        w611 = -1.0 ("default (0 DBL)")
        n178 = property on="String 2" class="Str"() -> ("Text.Text"=w613:string)  [unwired: 2 in, 2 out]
        n179 = Fract/Exp String To Number(use system decimal point (T)=TRUE, string=w613, default (0 dbl)=w611) -> (number=w612:dbl)  [unwired: 1 in, 1 out]
        n180 = Concatenate Strings("Operación: Depósito a ", "Combo Box 2", ", Cantidad Donada: $") -> (w623:string)
        n181 = event shown="[13] \"Boton_Aceptar\": Value Change" {
          selector: _ -> [_ _ _ _ _ _ _ _ _ _ _ _ _ _ _]
          dyn-events: _ -> [_ _ _ _ _ _ _ _ _ _ _ _ _ _ _]
          timeout: _ -> [_ _ _ _ _ _ _ _ _ _ _ _ _ _ _]
          tunnel: [w637 w645 w653 w661 w669 w677 w685 w693 w701 w709 w717 w725 "" w739 w790] -> w614
          tunnel: [Control_1Enum."Depositos" Control_1Enum."Depositos" Control_1Enum."Depositos" Control_1Enum."Depositos" Control_1Enum."Depositos" Control_1Enum."Depositos" Control_1Enum."Depositos" Control_1Enum."Depositos" Control_1Enum."Depositos" Control_1Enum."Depositos" Control_1Enum."Depositos" Control_1Enum."Depositos" Control_1Enum."Depositos" w741 Control_1Enum."Menu_Principal"] -> w631
          tunnel: [u8 7 u8 7 u8 7 u8 7 u8 7 u8 7 u8 7 u8 7 u8 7 u8 7 u8 7 u8 7 u8 7 w740 u8 2] -> w630
          tunnel: w624 -> [w632 w641 w649 w657 w665 w673 w681 w689 w697 w705 w713 w721 w731 w755 w795]
          tunnel: w623 -> [_ _ _ _ _ _ _ _ _ _ _ _ _ w754 _]
          tunnel: ", Crédito Anterior: $" -> [_ _ _ _ _ _ _ _ _ _ _ _ _ w753 _]
          tunnel: w621 -> [w634 w642 w650 w658 w666 w674 w682 w690 w698 w706 w714 w722 w732 w752 w794]
          tunnel: ", Deuda Anterior: $" -> [_ _ _ _ _ _ _ _ _ _ _ _ _ w751 _]
          tunnel: w619 -> [w633 w640 w648 w656 w664 w672 w680 w688 w696 w704 w712 w720 w730 w750 w793]
          tunnel: ", Crédito Disponible: $" -> [_ _ _ _ _ _ _ _ _ _ _ _ _ w749 _]
          tunnel: ", Deuda: $" -> [_ _ _ _ _ _ _ _ _ _ _ _ _ w748 _]
          tunnel: "\r\n" -> [_ _ _ _ _ _ _ _ _ _ _ _ _ w747 _]
          tunnel: w612 -> [_ _ _ _ _ _ _ _ _ _ _ _ _ w742 _]
          tunnel: w611 -> [_ _ _ _ _ _ _ _ _ _ _ _ _ w746 _]
          tunnel: [w632 w641 w649 w657 w665 w673 w681 w689 w697 w705 w713 w721 w731 w738 w795] -> w610
          tunnel: [w634 w642 w650 w658 w666 w674 w682 w690 w698 w706 w714 w722 w732 w737 w794] -> w609
          tunnel: [w633 w640 w648 w656 w664 w672 w680 w688 w696 w704 w712 w720 w730 w736 w793] -> w608
          event "Boton_0": Value Change {
            # "Pantalla Depósitos"
            n182 = event-data() -> ()  [unwired: 1 in, 2 out]
            n183 = property on="String 2" class="Str"() -> ("Text.Text"=w639:string)  [unwired: 2 in, 2 out]
            n184 = Concatenate Strings(w639, "0") -> (w637:string)
          }
          event "Boton_1": Value Change {
            # "Pantalla Depósitos"
            n185 = event-data() -> ()  [unwired: 1 in, 2 out]
            n186 = property on="String 2" class="Str"() -> ("Text.Text"=w647:string)  [unwired: 2 in, 2 out]
            n187 = Concatenate Strings(w647, "1") -> (w645:string)
          }
          event "Boton_2": Value Change {
            # "Pantalla Depósitos"
            n188 = event-data() -> ()  [unwired: 1 in, 1 out]
            n189 = property on="String 2" class="Str"() -> ("Text.Text"=w655:string)  [unwired: 2 in, 2 out]
            n190 = Concatenate Strings(w655, "2") -> (w653:string)
          }
          event "Boton_3": Value Change {
            # "Pantalla Depósitos"
            n191 = event-data() -> ()  [unwired: 1 in, 2 out]
            n192 = property on="String 2" class="Str"() -> ("Text.Text"=w663:string)  [unwired: 2 in, 2 out]
            n193 = Concatenate Strings(w663, "3") -> (w661:string)
          }
          event "Boton_4": Value Change {
            # "Pantalla Depósitos"
            n194 = event-data() -> ()  [unwired: 1 in, 2 out]
            n195 = property on="String 2" class="Str"() -> ("Text.Text"=w671:string)  [unwired: 2 in, 2 out]
            n196 = Concatenate Strings(w671, "4") -> (w669:string)
          }
          event "Boton_5": Value Change {
            # "Pantalla Depósitos"
            n197 = event-data() -> ()  [unwired: 1 in, 2 out]
            n198 = property on="String 2" class="Str"() -> ("Text.Text"=w679:string)  [unwired: 2 in, 2 out]
            n199 = Concatenate Strings(w679, "5") -> (w677:string)
          }
          event "Boton_6": Value Change {
            # "Pantalla Depósitos"
            n200 = event-data() -> ()  [unwired: 1 in, 2 out]
            n201 = property on="String 2" class="Str"() -> ("Text.Text"=w687:string)  [unwired: 2 in, 2 out]
            n202 = Concatenate Strings(w687, "6") -> (w685:string)
          }
          event "Boton_7": Value Change {
            # "Pantalla Depósitos"
            n203 = event-data() -> ()  [unwired: 1 in, 2 out]
            n204 = property on="String 2" class="Str"() -> ("Text.Text"=w695:string)  [unwired: 2 in, 2 out]
            n205 = Concatenate Strings(w695, "7") -> (w693:string)
          }
          event "Boton_8": Value Change {
            # "Pantalla Depósitos"
            n206 = event-data() -> ()  [unwired: 1 in, 2 out]
            n207 = property on="String 2" class="Str"() -> ("Text.Text"=w703:string)  [unwired: 2 in, 2 out]
            n208 = Concatenate Strings(w703, "8") -> (w701:string)
          }
          event "Boton_9": Value Change {
            # "Pantalla Depósitos"
            n209 = event-data() -> ()  [unwired: 1 in, 6 out]
            n210 = property on="String 2" class="Str"() -> ("Text.Text"=w711:string)  [unwired: 2 in, 2 out]
            n211 = Concatenate Strings(w711, "9") -> (w709:string)
          }
          event "Boton_Punto": Value Change {
            # "Pantalla Depósitos"
            n212 = event-data() -> ()  [unwired: 1 in, 6 out]
            n213 = property on="String 2" class="Str"() -> ("Text.Text"=w719:string)  [unwired: 2 in, 2 out]
            n214 = Concatenate Strings(w719, ".") -> (w717:string)
          }
          event "Boton_Borrar": Value Change {
            # "Pantalla Depósitos"
            n215 = event-data() -> ()  [unwired: 1 in, 6 out]
            n216 = property on="String 2" class="Str"() -> ("Text.Text"=w726:string)  [unwired: 2 in, 2 out]
            n217 = String Length(string=w726) -> (length=w723:i32)
            n218 = Decrement(x=w723) -> (x-1=w724:i32)
            n219 = String Subset(string=w726, offset (0)=0, length (rest)=w724) -> (substring=w725:string)
          }
          event "Boton_Limpiar": Value Change {
            # "Pantalla Depósitos"
            n220 = event-data() -> ()  [unwired: 1 in, 6 out]
          }
          event "Boton_Aceptar": Value Change {
            n221 = event-data() -> ()  [unwired: 1 in, 1 out]
            n222 = Greater Or Equal?(x=w752, y=w742) -> (x >= y?=w745:bool)
            n223 = Greater?(x=w742, y=w746) -> (0:w744:bool)
            n224 = And(x=w745, y=w744) -> (x .and. y?=w743:bool)
            n225 = case shown="True" w743 {
              tunnel: [w761 w788] -> w736
              tunnel: [w762 w785] -> w737
              tunnel: w752 -> [w762 w783]
              tunnel: w750 -> [w761 w781]
              tunnel: w755 -> [w763 w784]
              tunnel: w754 -> [_ w779]
              tunnel: w753 -> [_ w777]
              tunnel: w751 -> [_ w775]
              tunnel: w749 -> [_ w772]
              tunnel: w748 -> [_ w771]
              tunnel: w747 -> [_ w769]
              tunnel: [w763 w768] -> w738
              tunnel: w742 -> [_ w767]
              tunnel: [Control_1Enum."Depositos" Control_1Enum."Menu_Principal"] -> w741
              tunnel: [u8 7 u8 2] -> w740
              tunnel: [w758 ""] -> w739
              frame False {
                # "Pantalla Depósitos"
                n226 = property on="String 2" class="Str"() -> ("Text.Text"=w758:string)  [unwired: 2 in, 2 out]
                n227 = One Button Dialog(message="Datos Inválidos", button name ("OK")="Aceptar") -> ()  [unwired: 1 out]
              }
              frame True {
                # "P. Principal"
                n228 = Subtract(x=w783, y=w767) -> (x-y=w785:dbl)
                n229 = Add(x=w767, y=w781) -> (x+y=w788:dbl)
                n230 = Number To Fractional String(number=w781, precision (6)=i16 2) -> (F-format string=w774:string)  [unwired: 2 in]
                n231 = Number To Fractional String(number=w783, precision (6)=i16 2) -> (F-format string=w776:string)  [unwired: 2 in]
                n232 = Number To Fractional String(number=w767, precision (6)=i16 2) -> (F-format string=w778:string)  [unwired: 2 in]
                n233 = Number To Fractional String(number=w785, precision (6)=i16 2) -> (F-format string=w773:string)  [unwired: 2 in]
                n234 = Number To Fractional String(number=w788, precision (6)=i16 2) -> (F-format string=w770:string)  [unwired: 2 in]
                n235 = Concatenate Strings(w784, w779, w778, w777, w776, w775, w774, w772, w773, w771, w770, w769) -> (w768:string)
              }
            }
          }
          event "Regresar_5": Value Change {
            # "Pantalla Principal"
            n236 = event-data() -> ()  [unwired: 1 in, 2 out]
            n237 = property on="String 2" class="Str"() -> ("Text.Text"=w790:string)  [unwired: 2 in, 2 out]
          }
        }
        "String 2" <- w614
        "Credito_Disponible 6" <- w621
        "Adeudo_Tarjeta 6" <- w619
      }
      frame "Estado_Cuenta" {
        n238 = event shown="[1] \"Regresar_6\": Value Change" {
          selector: _ -> [_ _]
          dyn-events: _ -> [_ _]
          timeout: _ -> [_ _]
          tunnel: [_ Control_1Enum."Menu_Principal"] -> w799
          tunnel: [_ u8 2] -> w798
          tunnel: w797 -> [_ w804]
          tunnel: [_ w804] -> w796
          event Timeout {
            n239 = event-data() -> ()  [unwired: 1 in, 3 out]
          }
          event "Regresar_6": Value Change {
            # "Pantalla Principal"
            n240 = event-data() -> ()  [unwired: 1 in, 6 out]
          }
        }
        "Transacciones" <- w797
      }
    }
    "Tab Control" <- w24
    "String" <- w12
  }
